vi "Init Error Log.vi"(7 "TopLevel":refnum<vi>, 8 "error in (no error)":errorcluster, 9 "size(512kB)":u32(ring)=512 items=["125 kB"=125, "256 kB"=256, "512 kB"=512, "1024 kB"=1024, "2048 kB"=2048, "4096 kB"=4096, "8196 kB"=8196, "16384 kB"=16384, "32768 kB"=32768], 10 "Name(App)":string="App", 11 "LogRotate in":refnum<class "LogRotate.lvclass">) -> (0 "error out":errorcluster, 3 "LogRotate out":refnum<class "LogRotate.lvclass">)   [LabVIEW 2021, in "Error_Manager.lvlib" / "LogRotate.lvclass"]
uses:
  LogRotate.lvclass
  LogData.ctl
  LogRotate.lvclass/LogRotate.ctl
  Error Handler Queue.vi
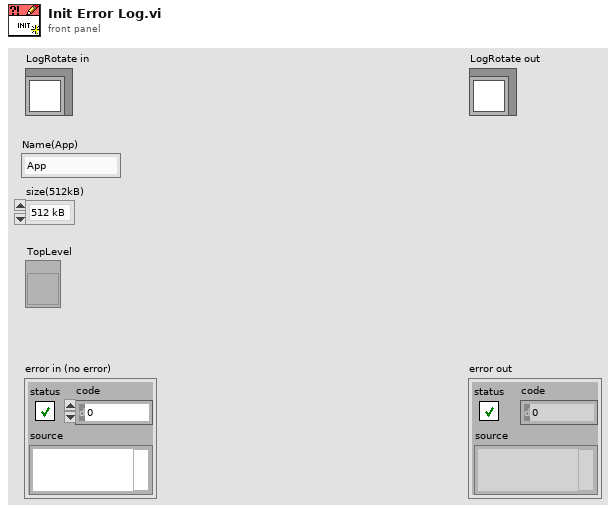
[diagram p1: front panel]
types:
  T1 = typedef "Error_Manager.lvlib/LogRotate.lvclass/LogData.ctl" = cluster{"error in":errorcluster, "replacements":string[], "Time Stamp":timestamp}
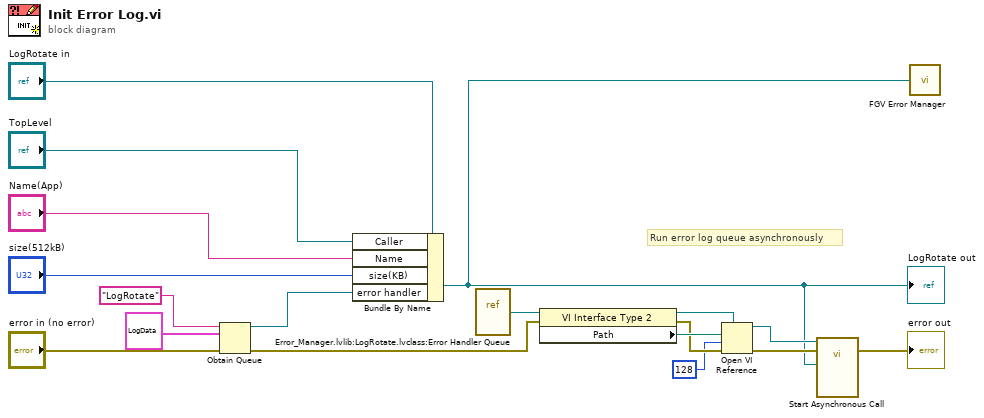
[diagram p0: block diagram]
diagram:
  # "Run error log queue asynchronously"
  n1 = Obtain Queue(name (unnamed)="LogRotate", element data type=T1 {"error in"={"status"=FALSE, "code"=0, "source"=""}, "replacements"=[], "Time Stamp"=timestamp(0 s since 1904-01-01)} ("LogData"), error in (no error)="error in (no error)") -> (queue out=w14:refnum<queue>, error out=w3:errorcluster)  [unwired: 2 in, 1 out]
  n2 = Bundle By Name(cluster="LogRotate in", "Caller"="TopLevel", "Name"="Name(App)", "size(KB)"="size(512kB)", "error handler"=w14) -> (w4:refnum<class "LogRotate.lvclass">)
  "LogRotate out" <- w4
  n3 = vi-ref "Error_Manager.lvlib:LogRotate.lvclass:Error Handler Queue.vi"() -> (w9:refnum<vi>)
  n4 = property class="VI Interface Type 2"(reference=w9, error in=w3) -> (reference out=w8:refnum<vi>, error out=w2:errorcluster, "Path"=w7:path)
  n5 = Open VI Reference(type specifier VI Refnum (for type only)=w8, vi path=w7, options=128, error in (no error)=w2) -> (vi reference=w5:refnum<vi>, error out=w10:errorcluster)  [unwired: 2 in]
  n6 = call-by-ref "Start Asynchronous Call"(reference=w5, error in=w10, "LogRotate in"=w4) -> (error out=→"error out":errorcluster)  [unwired: 10 in, 2 out]
  n7 = call "FGV Error Manager.vi"("error_manager in"=w4) -> ()  [unwired: 1 out]
